vi "Bridge Measure Single.vi"(7 "allow uncertainty calculation (true)":bool=TRUE, 8 "error in":errorcluster, 9 "stop ref (none)":refnum<vi>, 10 "sampling":T4, 11 "bridge in":T5={"type"=enum."TWM client", "TWM"={"pipe name"="", "parameters"=[], "handle"=0, "fixed aper [s]"=0.0, "f-list [Hz]"=[], "discrete f-list"=FALSE, "unc mode"=enum."None", "unc mcc"=0, "unc first"=FALSE, "alg id"=enum."TWM-LowZ - Low Z measurement"}, "last f"=0.0, "bias comp"={"bias type"=enum."dummy", "VISA"="", "Enable"=FALSE, "channel qu"=[], "channel Uinit"=[]}, "sim mode"=enum."Generic RLC network", "channel idns"=[], "sim phases"=1} {"TWM"."f-list [Hz]" format="%#_6p"}) -> (0 "error out":errorcluster, 1 "stoped?":bool, 2 "reading per phase":T1[](array[typedef]), 3 "bridge out":T5={"type"=enum."TWM client", "TWM"={"pipe name"="", "parameters"=[], "handle"=0, "fixed aper [s]"=0.0, "f-list [Hz]"=[], "discrete f-list"=FALSE, "unc mode"=enum."None", "unc mcc"=0, "unc first"=FALSE, "alg id"=enum."TWM-LowZ - Low Z measurement"}, "last f"=0.0, "bias comp"={"bias type"=enum."dummy", "VISA"="", "Enable"=FALSE, "channel qu"=[], "channel Uinit"=[]}, "sim mode"=enum."Generic RLC network", "channel idns"=[], "sim phases"=1} {"TWM"."f-list [Hz]" format="%#_6p"})   [LabVIEW 2020]
doc: "Setup bridge parameters."
uses:
  Bridge Session.ctl
  Bridge Type.ctl
  drivers/TWM client/TWM Session.ctl
  drivers/TWM client/TWM parameters.ctl
  drivers/TWM client/Meas Proc QWTB Uncertainty Mode.ctl
  Bridge Algorithm.ctl
  Bridge Bias Session.ctl
  Bridge Bias Type.ctl
  Bridge Sim Mode.ctl
  Bridge Sampling Setup.ctl
  Bridge Reading Data.ctl
  drivers/TWM client/Meas Proc QWTB Spectrum Data.ctl
  drivers/TWM client/TWM Phase Info.ctl
  drivers/TWM client.lvlibp/server/TWM client/TWM Client Result Max Dim.ctl
  drivers/TWM client.lvlibp/server/TWM client/TWM Client Quantity Record.ctl
  <vilib>/Analysis/baseanly.llb/Mean (DBL).vi
  drivers/TWM client.lvlibp
  <vilib>/Analysis/NI_AALBase.lvlib
panel:
  out "fake phase index":u16(ring)
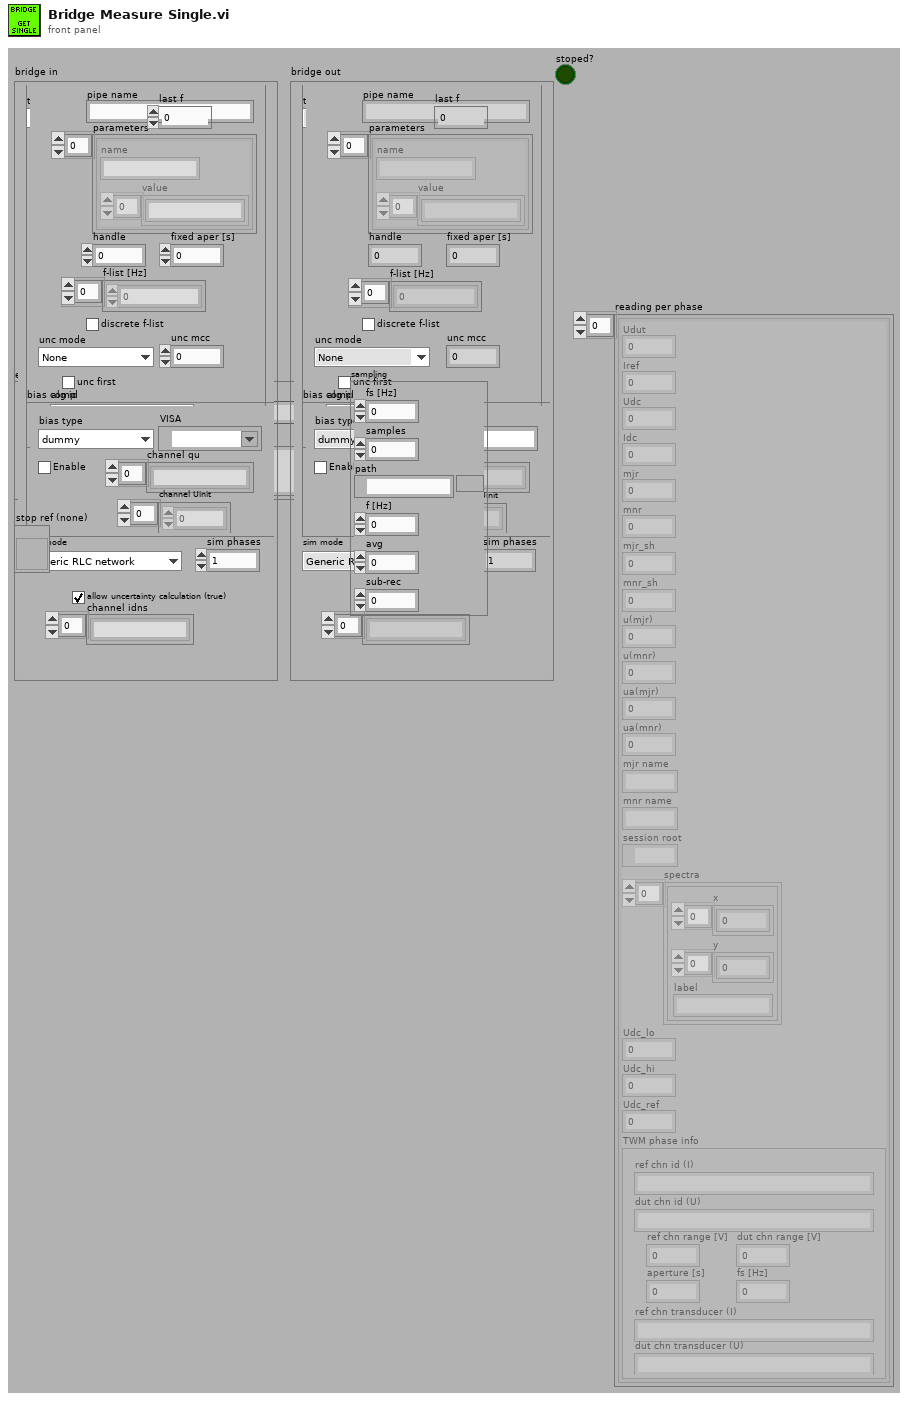
[diagram p1: front panel]
types:
  T1 = typedef "Bridge Reading Data.ctl" = cluster{"Udut":dbl, "Iref":dbl, "Udc":dbl, "Idc":dbl, "mjr":dbl, "mnr":dbl, "mjr_sh":dbl, "mnr_sh":dbl, "u(mjr)":dbl, "u(mnr)":dbl, "ua(mjr)":dbl, "ua(mnr)":dbl, "mjr name":string, "mnr name":string, "session root":path, "spectra":T2[], "Udc_lo":dbl, "Udc_hi":dbl, "Udc_ref":dbl, "TWM phase info":T3}
  T2 = typedef "Meas Proc QWTB Spectrum Data.ctl" = cluster{"x":sgl[], "y":sgl[], "label":string}
  T3 = typedef "TWM Phase Info.ctl" = cluster{"ref chn id (I)":string, "dut chn id (U)":string, "ref chn range [V]":dbl, "dut chn range [V]":dbl, "aperture [s]":dbl, "fs [Hz]":dbl, "ref chn transducer (I)":string, "dut chn transducer (U)":string}
  T4 = typedef "Bridge Sampling Setup.ctl" = cluster{"fs [Hz]":dbl, "samples":i32, "path":path, "f [Hz]":dbl, "avg":i32, "sub-rec":i32}
  T5 = typedef "Bridge Session.ctl" = cluster{"type":T6, "TWM":T7, "last f":dbl, "bias comp":T11, "sim mode":T13, "channel idns":string[], "sim phases":i32}
  T6 = typedef "Bridge Type.ctl" = enum16{"TWM client", "dummy"}
  T7 = typedef "TWM Session.ctl" = cluster{"pipe name":string, "parameters":T8[], "handle":i32, "fixed aper [s]":dbl, "f-list [Hz]":dbl[], "discrete f-list":bool, "unc mode":T9, "unc mcc":i32, "unc first":bool, "alg id":T10}
  T8 = typedef "TWM parameters.ctl" = cluster{"name":string, "value":string[]}
  T9 = typedef "Meas Proc QWTB Uncertainty Mode.ctl" = enum16{"None", "GUF", "Monte Carlo"}
  T10 = typedef "Bridge Algorithm.ctl" = enum16{"TWM-LowZ - Low Z measurement", "TWM-InpZ - Digitizer input Z measurement"}
  T11 = typedef "Bridge Bias Session.ctl" = cluster{"bias type":T12, "VISA":refnum<visa-resource-name>, "Enable":bool, "channel qu":string[], "channel Uinit":dbl[]}
  T12 = typedef "Bridge Bias Type.ctl" = enum16{"dummy", "CMI LiBbias V1.0"}
  T13 = typedef "Bridge Sim Mode.ctl" = enum16{"Generic RLC network", "Interchannel transfer", "Input impedance"}
  T14 = typedef "TWM client.lvlibp/TWM Client Result Max Dim.ctl" = enum16{"Scalar", "Vector", "Matrix"}
  T15 = typedef "TWM client.lvlibp/TWM Client Quantity Record.ctl" = cluster{"val":dbl[], "unc":dbl[], "name":string, "is valid?":bool, "has unc?":bool, "numel":i32, "ua":dbl[]}
  T16 = typedef "TWM client.lvlibp/TWM Client Result Info.ctl" = cluster{"qu. names":string[], "readings":i32, "qu. count":i32, "session root":string, "phase count":i32}
  T17 = typedef "TWM Session Data.ctl" = cluster{"digitizer channels":string[], "aux instruments":string[], "ranges [V]":dbl[], "apertures [s]":dbl[], "Ts [s]":dbl[], "mean apertures [s]":dbl, "mean fs [Hz]":dbl, "transducer paths":path[], "transducer is ref":bool[], "transducer phase":i32[], "transducer channel":i32[][], "transducer names":string[]}
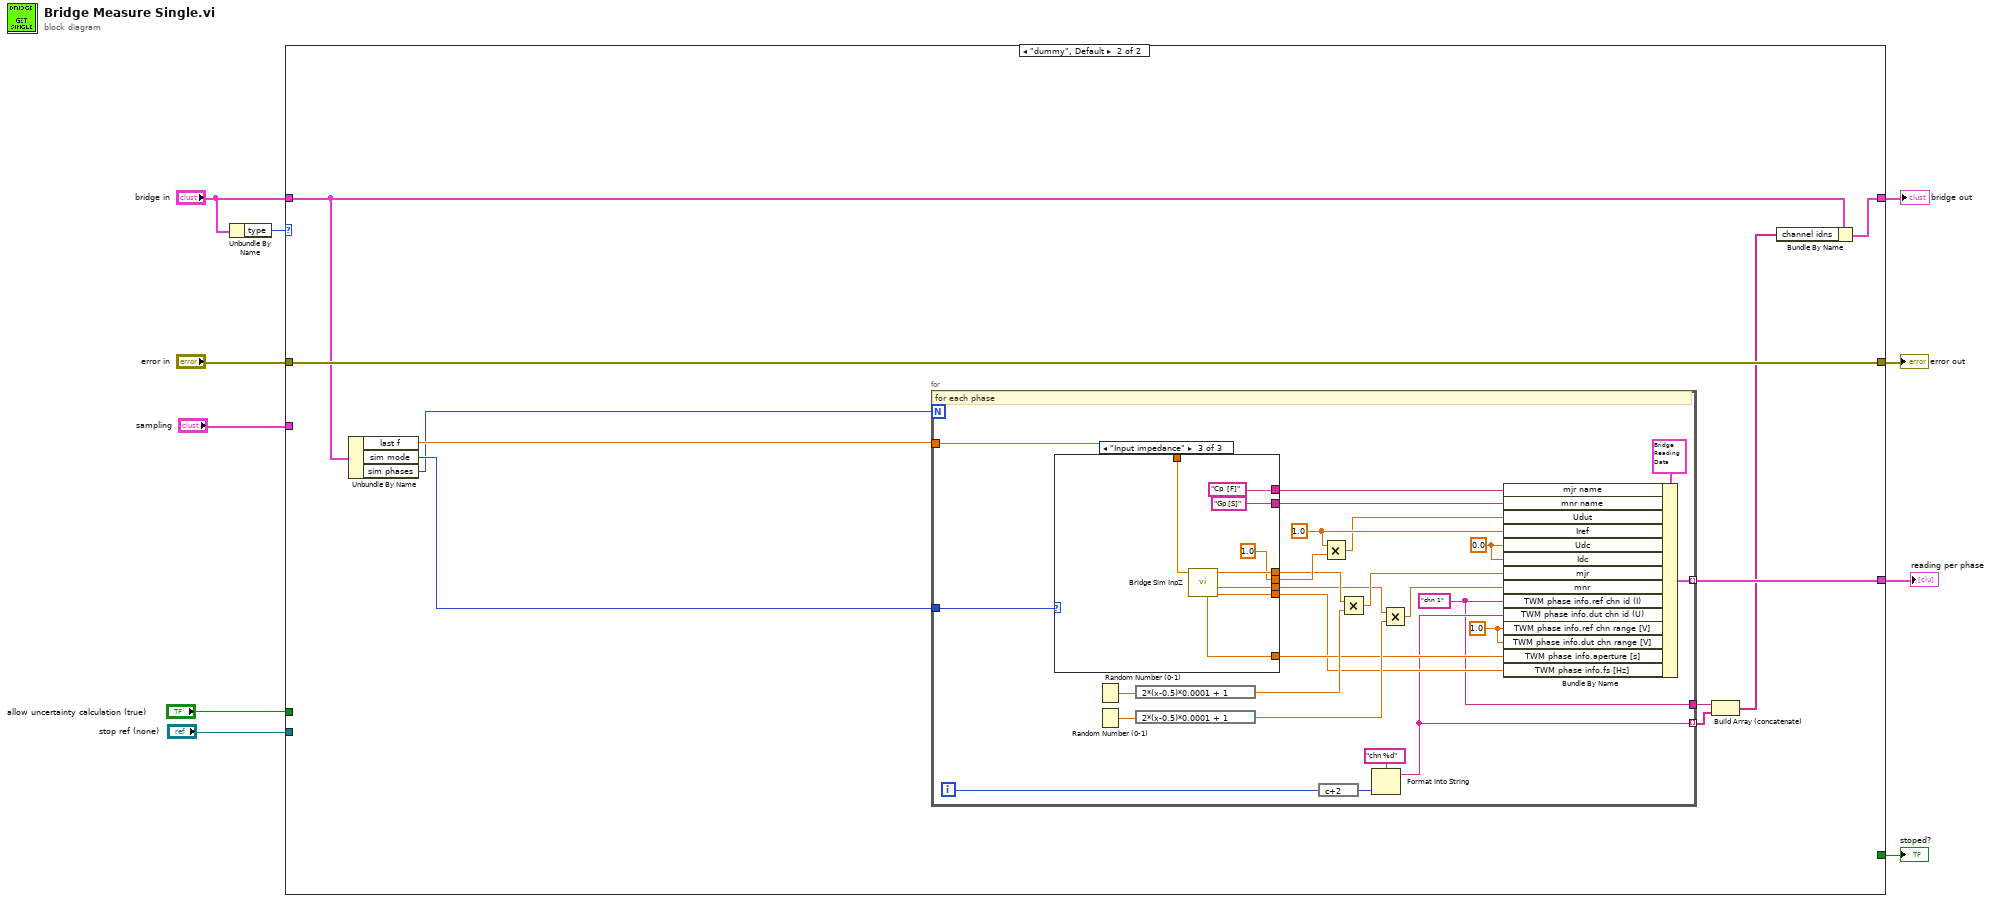
[diagram p0: block diagram]
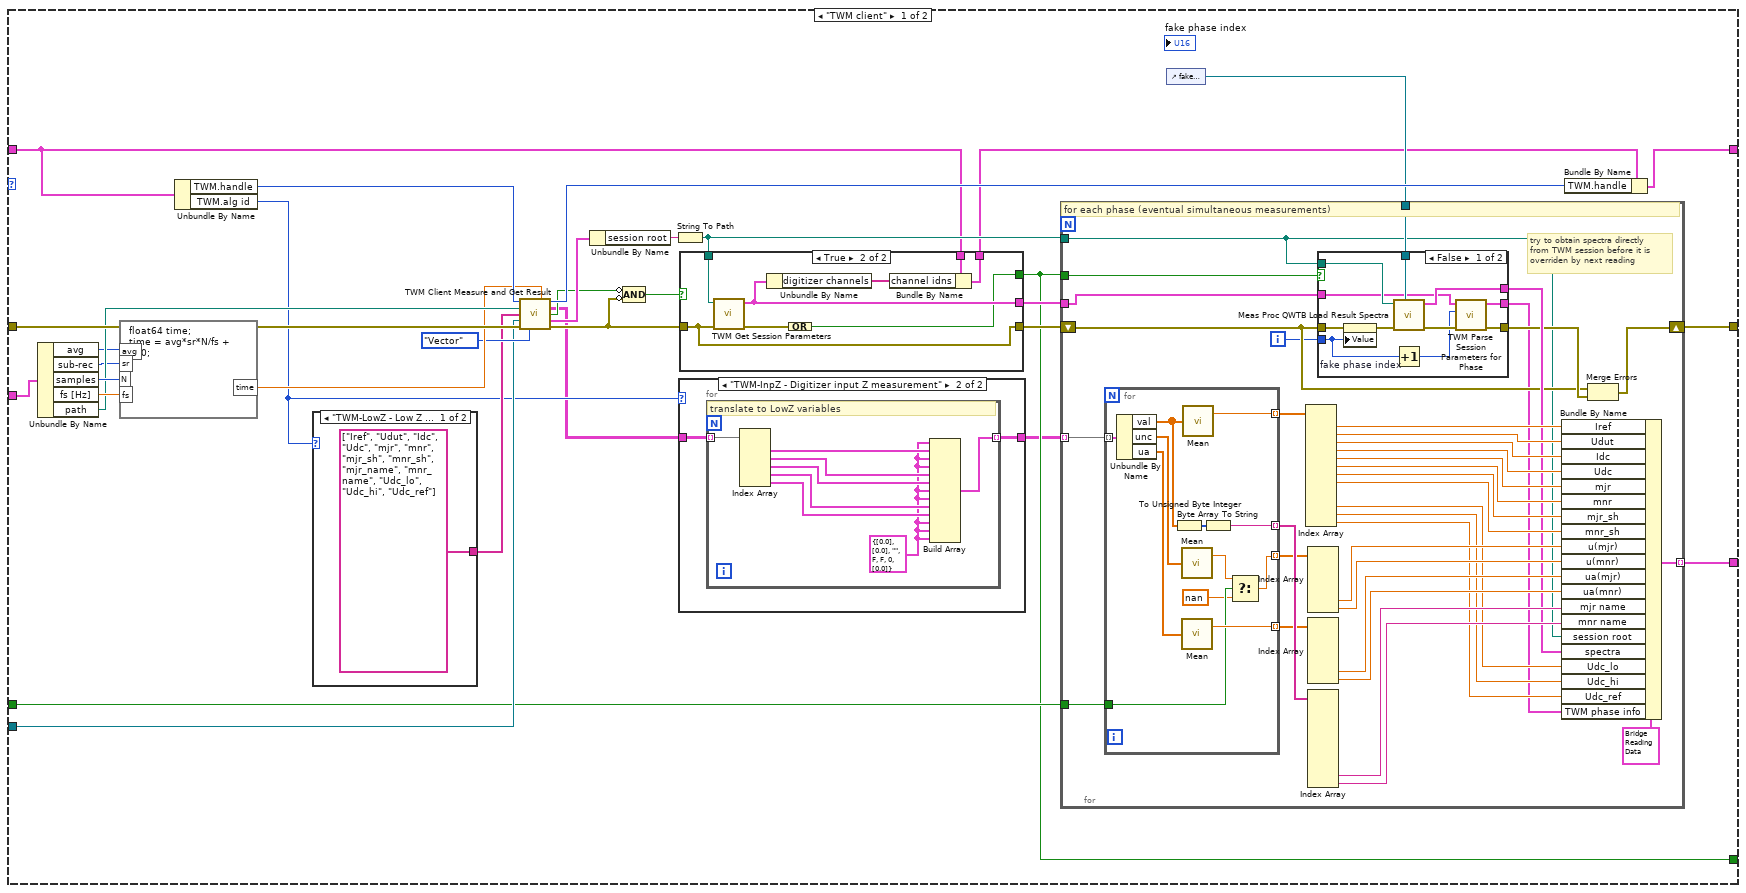
[diagram p2: hidden frame]
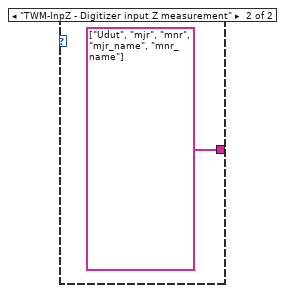
[diagram p4: hidden frame]
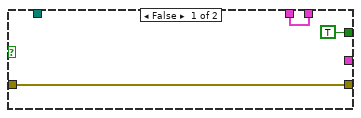
[diagram p5: hidden frame]
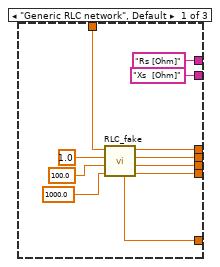
[diagram p7: hidden frame]
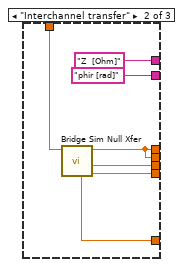
[diagram p8: hidden frame]
diagram:
  n1 = Unbundle By Name("bridge in") -> ("type"=w10:T6)
  n2 = case shown="\"dummy\", Default" w10 {
    tunnel: "error in" -> [w40 w135]
    tunnel: [w28 w135] -> w8
    tunnel: "bridge in" -> [w21 w130]
    tunnel: [w42 w129] -> w6
    tunnel: "sampling" -> [w41 _]
    tunnel: [w31 w132] -> w1
    tunnel: "stop ref (none)" -> [w29 _]
    tunnel: [w16 _] -> w3
    tunnel: "allow uncertainty calculation (true)" -> [w27 _]
    frame "TWM client" {
      n3 = Unbundle By Name(w41) -> ("avg"=w15:i32, "sub-rec"=w14:i32, "samples"=w38:i32, "fs [Hz]"=w37:dbl, "path"=w36:path)
      n4 = formula code="float64 time;\ntime = avg*sr*N/fs + 120;"("N"=w38, "fs"=w37, "avg"=w15, "sr"=w14) -> ("time"=w35:dbl)
      n5 = Unbundle By Name(w21) -> ("TWM.handle"=w39:i32, "TWM.alg id"=w13:T10)
      n6 = case shown="\"TWM-LowZ - Low Z measurement\", Default" w13 {
        tunnel: [string[] ["Iref", "Udut", "Idc", "Udc", "mjr", "mnr", "mjr_sh", "mnr_sh", "mjr_name", "mnr_name", "Udc_lo", "Udc_hi", "Udc_ref"] ("quantity names (all)") string[] ["Udut", "mjr", "mnr", "mjr_name", "mnr_name"] ("quantity names (all)")] -> w32
        frame "TWM-LowZ - Low Z measurement", Default {
        }
        frame "TWM-InpZ - Digitizer input Z measurement" {
        }
      }
      n7 = call "TWM Client Measure and Get Result.vi"("handle"=w39, "timeout [s] (10s)"=w35, "meas root path (last)"=w36, "quantity names (all)"=w32, "stop ref (none)"=w29, "error in"=w40, "qwtb maxdim (scalar)"=TWM_Client_Result_Max_Dim."Vector") -> ("handle out"=w33:i32, "data"=w11:T15[][], "stoped?"=w18:bool, "quantities"=w24:T16, "error out"=w19:errorcluster)  [unwired: 4 in]
      n8 = Unbundle By Name(w24) -> ("session root"=w25:string)
      n9 = Compound Arithmetic op=AND(invert w18, invert w19) -> (w17:bool)
      n10 = String To Path(string=w25) -> (path=w23:path)
      n11 = case shown="\"TWM-InpZ - Digitizer input Z measurement\"" w13 {
        tunnel: w11 -> [w43 w45]
        tunnel: [w43 w44] -> w12
        frame "TWM-LowZ - Low Z measurement", Default {
        }
        frame "TWM-InpZ - Digitizer input Z measurement" {
          n12 = for {
            tunnel: w45 -> [w53] mode=indexing
            tunnel: [w47] -> w44 mode=indexing
            w46 = T15 {"val"=[0.0], "unc"=[0.0], "name"="", "is valid?"=FALSE, "has unc?"=FALSE, "numel"=0, "ua"=[0.0]} ("quantity")
            # "translate to LowZ variables"
            n13 = Index Array(array=w53) -> (element #1=w52:T15, element #2=w51:T15, element #3=w50:T15, element #4=w49:T15, element #5=w48:T15)  [unwired: 5 in]
            n14 = Build Array(w46, w52, w46, w46, w51, w50, w46, w46, w49, w48, w46, w46, w46) -> (w47:T15[])
          }
        }
      }
      n15 = case shown="True" w17 {
        tunnel: w19 -> [w58 w59]
        tunnel: [w58 w59] -> w26
        tunnel: w23 -> [_ w66]
        tunnel: [_ w65] -> w22
        tunnel: w21 -> [w57 w64]
        tunnel: [w57 w63] -> w20
        tunnel: [TRUE w60] -> w16
        frame False {
        }
        frame True {
          n16 = call "TWM Get Session Parameters.vi"("error in"=w59, "meas root"=w66) -> ("error out"=w61:errorcluster, "TWM session items"=w65:T17)  [unwired: 7 in, 1 out]
          n17 = Unbundle By Name(w65) -> ("digitizer channels"=w62:string[])
          n18 = Compound Arithmetic op=OR(w61) -> (w60:bool)
          n19 = Bundle By Name(cluster=w64, "channel idns"=w62) -> (w63:T5)
        }
      }
      n20 = control-ref of="fake phase index"() -> (w30:refnum<vi>)
      n21 = for {
        tunnel: [w93] -> w31 mode=indexing
        tunnel: w12 -> [w71] mode=indexing
        tunnel: w30 -> [w80]
        tunnel: w16 -> [w77]
        tunnel: w27 -> [w76]
        shift-right: [w78] -> w28
        shift-left: w26 -> [w72]
        tunnel: w23 -> [w69]
        tunnel: w22 -> [w68]
        i -> [w70]
        # "try to obtain spectra directly\nfrom TWM session before it is\noverriden by next reading"
        # "for each phase (eventual simultaneous measurements)"
        n22 = for {
          tunnel: w71 -> [w125] mode=indexing
          tunnel: [w124] -> w101 mode=indexing
          tunnel: [w121] -> w92 mode=indexing
          tunnel: [w114] -> w91 mode=indexing
          tunnel: [w118] -> w90 mode=indexing
          tunnel: w76 -> [w117]
          n23 = Unbundle By Name(w125) -> ("val"=w123:dbl[], "unc"=w120:dbl[], "ua"=w119:dbl[])
          n24 = To Unsigned Byte Integer(number=w123) -> (unsigned 8bit integer=w122:u8[])
          n25 = call-poly <vilib>:"Mean.vi"("X"=w120) -> ("mean"=w116:dbl)  [unwired: 1 out]
          n26 = call-poly <vilib>:"Mean.vi"("X"=w119) -> ("mean"=w118:dbl)  [unwired: 1 out]
          n27 = call-poly <vilib>:"Mean.vi"("X"=w123) -> ("mean"=w124:dbl)  [unwired: 1 out]
          n28 = Byte Array To String(unsigned byte array=w122) -> (string=w121:string)
          n29 = Select(t=w116, s=w117, f=nan) -> (s? t:f=w114:dbl)
        }
        n30 = Index Array(array=w101) -> (element #1=w99:dbl, element #2=w98:dbl, element #3=w97:dbl, element #4=w96:dbl, element #5=w95:dbl, element #6=w94:dbl, element #7=w85:dbl, element #8=w84:dbl, element #11=w75:dbl, element #12=w74:dbl, element #13=w73:dbl)  [unwired: 13 in, 2 out]
        n31 = Index Array(array=w91) -> (element #5=w89:dbl, element #6=w88:dbl)  [unwired: 6 in, 4 out]
        n32 = Index Array(array=w90) -> (element #5=w87:dbl, element #6=w86:dbl)  [unwired: 6 in, 4 out]
        n33 = Index Array(array=w92) -> (element #9=w82:string, element #10=w83:string)  [unwired: 10 in, 8 out]
        n34 = case shown="False" w77 {
          tunnel: w69 -> [w108 _]
          tunnel: [w112 _] -> w81
          tunnel: w80 -> [w111 _]
          tunnel: w72 -> [w109 w113]
          tunnel: [w106 w113] -> w79
          tunnel: w70 -> [w104 _]
          tunnel: w68 -> [w105 _]
          tunnel: [w102 _] -> w67
          frame False {
            n35 = property on="fake phase index" class="Ring (strict)"(error in=w109, "Value"=w104) -> (error out=w110:errorcluster)  [unwired: 1 in, 1 out]
            n36 = call "Meas Proc QWTB Load Result Spectra.vi"("phase ref"=w111, "error in"=w110, "meas root"=w108) -> ("error out"=w107:errorcluster, "graphs"=w112:T2[])  [unwired: 7 in]
            n37 = Increment(x=w104) -> (x+1=w103:i32)
            n38 = call "TWM Parse Session Parameters for Phase.vi"("error in"=w107, "phase index (1: default)"=w103, "TWM session items"=w105) -> ("error out"=w106:errorcluster, "TWM channel info"=w102:T3)  [unwired: 7 in]
          }
          frame True {
          }
        }
        n39 = Bundle By Name(cluster=T1 {"Udut"=0.0, "Iref"=0.0, "Udc"=0.0, "Idc"=0.0, "mjr"=0.0, "mnr"=0.0, "mjr_sh"=0.0, "mnr_sh"=0.0, "u(mjr)"=0.0, "u(mnr)"=0.0, "ua(mjr)"=0.0, "ua(mnr)"=0.0, "mjr name"="", "mnr name"="", "session root"=path "", "spectra"=[], "Udc_lo"=0.0, "Udc_hi"=0.0, "Udc_ref"=0.0, "TWM phase info"={"ref chn id (I)"="", "dut chn id (U)"="", "ref chn range [V]"=0.0, "dut chn range [V]"=0.0, "aperture [s]"=0.0, "fs [Hz]"=0.0, "ref chn transducer (I)"="", "dut chn transducer (U)"=""}} ("reading"), "Iref"=w99, "Udut"=w98, "Idc"=w97, "Udc"=w96, "mjr"=w95, "mnr"=w94, "mjr_sh"=w85, "mnr_sh"=w84, "u(mjr)"=w89, "u(mnr)"=w88, "ua(mjr)"=w87, "ua(mnr)"=w86, "mjr name"=w82, "mnr name"=w83, "session root"=w69, "spectra"=w81, "Udc_lo"=w75, "Udc_hi"=w74, "Udc_ref"=w73, "TWM phase info"=w67) -> (w93:T1)
        n40 = Merge Errors(w72, w79) -> (w78:errorcluster)
      }
      n41 = Bundle By Name(cluster=w20, "TWM.handle"=w33) -> (w42:T5)
    }
    frame "dummy", Default {
      n42 = Unbundle By Name(w130) -> ("last f"=w134:dbl, "sim mode"=w133:T13, "sim phases"=w131:i32)
      n43 = for {
        N: w131 -> [_]
        tunnel: w134 -> [w160]
        tunnel: w133 -> [w144]
        tunnel: [w141] -> w132 mode=indexing
        tunnel: [w139] -> w127 mode=indexing
        tunnel: [w136] -> w128
        i -> [w138]
        w147 = 1.0 ("TWM phase info.ref chn range [V]")
        w136 = "chn 1" ("TWM phase info.ref chn id (I)")
        w156 = 0.0 ("Udc")
        w159 = 1.0 ("x")
        # "for each phase"
        n44 = case shown="\"Input impedance\"" w144 {
          tunnel: w160 -> [w172 w179 w187]
          tunnel: [w168 w175 1.0 ("x")] -> w158
          tunnel: [w167 w175 w183] -> w153
          tunnel: [w166 w178 w186] -> w151
          tunnel: [w165 w177 w185] -> w146
          tunnel: [w164 w176 w184] -> w145
          tunnel: ["Rs [Ohm]" ("mjr name") "Z  [Ohm]" ("mjr name") "Cp  [F]" ("mjr name")] -> w143
          tunnel: ["Xs  [Ohm]" ("mjr name") "phir [rad]" ("mjr name") "Gp [S]" ("mjr name")] -> w142
          frame "Generic RLC network", Default {
            n45 = call "RLC_fake.vi"("f [Hz]"=w172, "Rp [Ohm]"=1.0, "f1 [Hz]"=100.0, "f2 [Hz]"=1000.0 ("f1 [Hz]")) -> ("aperture"=w165:dbl, "Rs"=w167:dbl, "Z"=w168:dbl, "Xs"=w166:dbl, "fs"=w164:dbl)  [unwired: 1 in]
          }
          frame "Interchannel transfer" {
            n46 = call "Bridge Sim Null Xfer.vi"("f [Hz]"=w179) -> ("aperture"=w177:dbl, "gain"=w175:dbl, "phi"=w178:dbl, "fs"=w176:dbl)  [unwired: 5 in]
          }
          frame "Input impedance" {
            n47 = call "Bridge Sim InpZ.vi"("f [Hz]"=w187) -> ("aperture"=w185:dbl, "Cp"=w183:dbl, "Gp"=w186:dbl, "fs"=w184:dbl)  [unwired: 5 in]
          }
        }
        n48 = Random Number (0-1)() -> (number: 0 to 1=w155:dbl)
        n49 = Random Number (0-1)() -> (number: 0 to 1=w149:dbl)
        n50 = expression code="2*(x-0.5)*0.0001 + 1"(w155) -> (w154:dbl)
        n51 = expression code="2*(x-0.5)*0.0001 + 1"(w149) -> (w148:dbl)
        n52 = expression code="c+2"(w138) -> (w137:i32)
        n53 = Multiply(x=w159, y=w158) -> (x*y=w157:dbl)
        n54 = Multiply(x=w153, y=w154) -> (x*y=w152:dbl)
        n55 = Format Into String(format string="chn %d", w137) -> (resulting string=w139:string)  [unwired: 2 in, 1 out]
        n56 = Multiply(x=w151, y=w148) -> (x*y=w150:dbl)
        n57 = Bundle By Name(cluster=T1 {"Udut"=0.0, "Iref"=0.0, "Udc"=0.0, "Idc"=0.0, "mjr"=0.0, "mnr"=0.0, "mjr_sh"=0.0, "mnr_sh"=0.0, "u(mjr)"=0.0, "u(mnr)"=0.0, "ua(mjr)"=0.0, "ua(mnr)"=0.0, "mjr name"="", "mnr name"="", "session root"=path "", "spectra"=[], "Udc_lo"=0.0, "Udc_hi"=0.0, "Udc_ref"=0.0, "TWM phase info"={"ref chn id (I)"="", "dut chn id (U)"="", "ref chn range [V]"=0.0, "dut chn range [V]"=0.0, "aperture [s]"=0.0, "fs [Hz]"=0.0, "ref chn transducer (I)"="", "dut chn transducer (U)"=""}} ("reading"), "mjr name"=w143, "mnr name"=w142, "Udut"=w157, "Iref"=w159, "Udc"=w156, "Idc"=w156, "mjr"=w152, "mnr"=w150, "TWM phase info.ref chn id (I)"=w136, "TWM phase info.dut chn id (U)"=w139, "TWM phase info.ref chn range [V]"=w147, "TWM phase info.dut chn range [V]"=w147, "TWM phase info.aperture [s]"=w146, "TWM phase info.fs [Hz]"=w145) -> (w141:T1)
      }
      n58 = Build Array (concatenate)(w128, w127) -> (w126:string[])
      n59 = Bundle By Name(cluster=w130, "channel idns"=w126) -> (w129:T5)
    }
  }
  "error out" <- w8
  "bridge out" <- w6
  "stoped?" <- w3
  "reading per phase" <- w1
